vi "P612_Quit.vi"(11 "VISA Refnum in":refnum<visa-resource-name>) -> ()   [LabVIEW 2014]
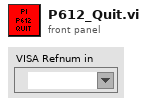
[diagram p1: front panel]
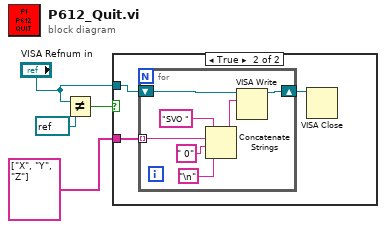
[diagram p0: block diagram]
diagram:
  n1 = Not Equal?(x="VISA Refnum in", y=refnum<visa-resource-name> refnum ("VISA resource name")) -> (x != y?=w2:bool)
  n2 = case shown="True" w2 {
    tunnel: "VISA Refnum in" -> [_ w7]
    tunnel: string[] ["X", "Y", "Z"] -> [_ w5]
    frame False {
    }
    frame True {
      n3 = for {
        shift-right: [w13] -> w6
        shift-left: w7 -> [w14]
        tunnel: w5 -> [w8] mode=indexing
        n4 = Concatenate Strings("SVO " ("write buffer"), w8, " 0" ("string"), "\n") -> (w11:string)
        n5 = VISA Write(VISA resource name=w14, write buffer=w11) -> (VISA resource name out=w13:refnum<visa-resource-name>)  [unwired: 1 in, 2 out]
      }
      n6 = VISA Close(VISA resource name=w6) -> ()  [unwired: 1 in, 1 out]
    }
  }
